vi "Post Build.vi"(0 "NIPKG_LV In":refnum<class "NIPKG_LV.lvclass">) -> (4 "NIPKG_LV out":refnum<class "NIPKG_LV.lvclass">)   [LabVIEW 2017, in "CL_G3_VIComponentBuilder.lvlib" / "NIPKG_LV.lvclass"]
doc: "Verifies that the built ni package was successfully registerd in the build machine feed."
uses:
  NIPKG_LV.lvclass
  C:/Tool Chain Support/Software Module Builder/Source/Exports/Exports/Export.lvclass
  Exports/Export.lvclass/Export.ctl
  <vilib>/Utility/sysdir.llb/System Directory Type.ctl
  Exports/Accessors/Read Built Version.vi
  Exports/Accessors/Read unique Name.vi
  Exports/Accessors/Write Export Operation Errors.vi
  Exports/Accessors/Read Export Operation Errors.vi
  NI Build Specification_LV/NI Build Specification_LV.lvclass
  <userlib>/_Cirrus Logic/NI Package Manager API/Source/TCS_NIPKG_API.lvlib
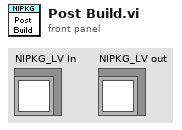
[diagram p1: front panel]
types:
  T1 = typedef "System Directory Type.ctl" = i32
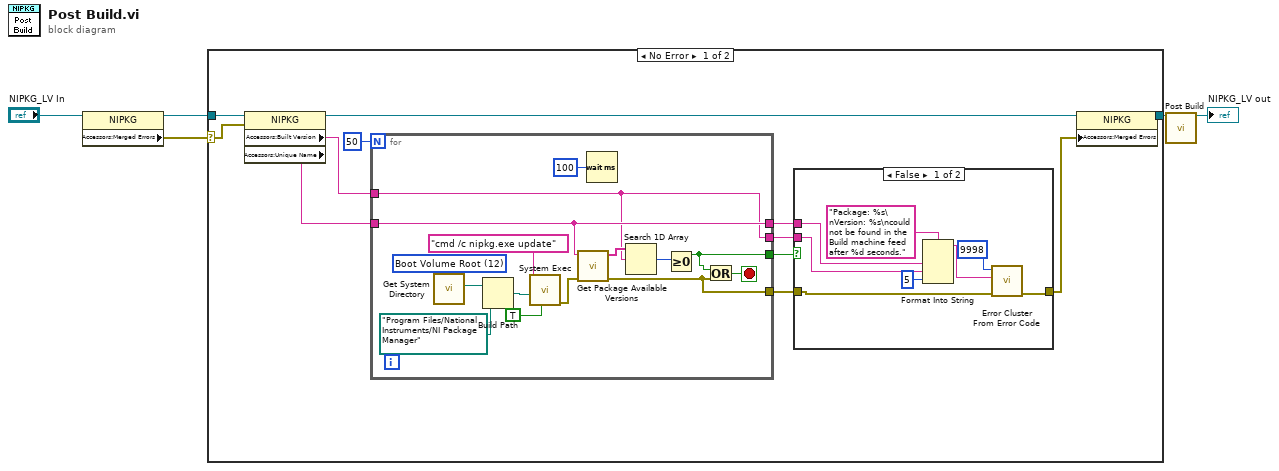
[diagram p0: block diagram]
diagram:
  n1 = property class="NIPKG"(reference="NIPKG_LV In") -> (reference out=w4:refnum<class "NIPKG_LV.lvclass">, "Accessors:Merged Errors"=w1:errorcluster)  [unwired: 1 in, 1 out]
  n2 = case shown="No Error" w1 {
    selector: w1 -> [w6 _]
    tunnel: w4 -> [w17 w42]
    tunnel: [w8 w42] -> w2
    frame No Error {
      n3 = property class="NIPKG"(reference=w17, error in=w6) -> (reference out=w9:refnum<class "NIPKG_LV.lvclass">, "Accessors:Built Version"=w15:string, "Accessors:Unique Name"=w14:string)  [unwired: 1 out]
      n4 = for {
        N: 50 -> [_]
        tunnel: w15 -> [w27]
        tunnel: w14 -> [w31]
        tunnel: [w32] -> w12
        tunnel: [w28] -> w13
        tunnel: [w31] -> w11
        tunnel: [w27] -> w10
        stop <- w33 stop-if-true
        w37 = T1 12 items=["User Home"=0, "User Desktop"=1, "User Documents"=2, "User Application Data"=3, "User Preferences"=4, "User Temporary"=5, "Public Documents"=6, "Public Application Data"=7, "Public Preferences"=8, "Public Cache"=13, "System Core Libraries"=9, "System Installed Libraries"=10, "Application Files"=11, "Boot Volume Root"=12] ("system directory type")
        # "Wait until the cache is refreshed"
        n5 = call <vilib>:"Get System Directory.vi"("system directory type"=w37) -> ("system directory"=w39:path)  [unwired: 10 in]
        n6 = Build Path(base path=w39, name or relative path=path "Program Files/National Instruments/NI Package Manager" ("working directory")) -> (appended path=w40:path)
        n7 = call <vilib>:"System Exec.vi"("run minimized? (F)"=TRUE, "working directory"=w40, "command line"="cmd /c nipkg.exe update" ("format string")) -> ("error out"=w34:errorcluster)  [unwired: 5 in, 3 out]
        n8 = call <userlib>:"Get Package Available Versions.vi"("error in"=w34, "package name"=w31) -> ("error out"=w32:errorcluster, "Versions"=w30:string[])  [unwired: 8 in]
        n9 = Wait (ms)(milliseconds to wait=u32 100) -> ()  [unwired: 1 out]
        n10 = Search 1D Array(1D array=w30, element=w27) -> (index of element=w29:i32)  [unwired: 1 in]
        n11 = Greater Or Equal To 0?(x=w29) -> (x >= 0?=w28:bool)
        n12 = Or(x=w28, y=w32) -> (x .or. y?=w33:bool)
      }
      n13 = case shown="False" w13 {
        tunnel: w12 -> [w25 w26]
        tunnel: [w24 w26] -> w7
        tunnel: w11 -> [w20 _]
        tunnel: w10 -> [w19 _]
        frame False {
          n14 = Format Into String(format string="Package: %s\nVersion: %s\ncould not be found in the Build machine feed after %d seconds.", w20, w19, 5 ("input 3")) -> (resulting string=w22:string)  [unwired: 2 in, 1 out]
          n15 = call <vilib>:"Error Cluster From Error Code.vi"("error in (no error)"=w25, "error message (\"\")"=w22, "error code (0)"=9998) -> ("error out"=w24:errorcluster)  [unwired: 6 in]
        }
        frame True {
        }
      }
      n16 = property class="NIPKG"(reference=w9, "Accessors:Merged Errors"=w7) -> (reference out=w8:refnum<class "NIPKG_LV.lvclass">)  [unwired: 1 in, 1 out]
    }
    frame Error {
    }
  }
  n17 = call-parent "Post Build.vi"("Export In"=w2) -> ("Export out"=→"NIPKG_LV out":refnum<class "NIPKG_LV.lvclass">)  [unwired: 14 in]
